vi "Create.vi"(8 "error in (no error)":errorcluster, 11 "GPIO #":T1=-1) -> (0 "error out":errorcluster, 3 "GPIO out":refnum<class "GPIO.lvclass">)   [LabVIEW 2020, in "CTI.lvlib" / "GPIO.lvclass"]
uses:
  GPIO.lvclass
  GPIO Number.ctl
  GPIO.lvclass/GPIO.ctl
  CTI.lvlib
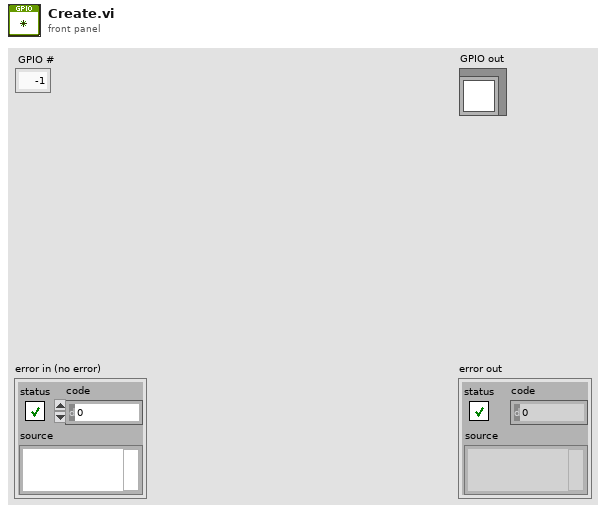
[diagram p1: front panel]
types:
  T1 = typedef "CTI.lvlib/GPIO Number.ctl" = i8
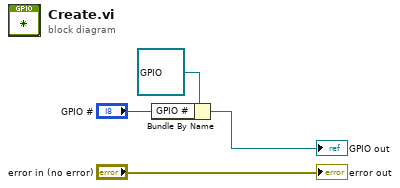
[diagram p0: block diagram]
diagram:
  n1 = Bundle By Name(cluster=refnum<class "GPIO.lvclass"> refnum ("GPIO in"), "GPIO #"="GPIO #") -> (→"GPIO out":refnum<class "GPIO.lvclass">)
  "error out" <- "error in (no error)"
